vi "I64_Write.vi"(8 "error in (no error)":errorcluster, 9 "Value":i64, 11 "Tag Name":string) -> (0 "error out":errorcluster)   [LabVIEW 2010, in "Current Value Table.lvlib"]
doc: "This VI will write the data associated with a single tag. This VI will always look up the tag index if the name changes, or if index lookup failed previously (resulting in an error). This combines the functionality of the CVT2 VIs for writes and static writes."
uses:
  Current Value Table.lvlib
  FGVs/Tag Memory Methods.ctl
  Type Defs/Memory Commands.ctl
  I64_Type To Enum.vi
  FGVs/CVT Globals.vi
  I64_Memory Block.vi
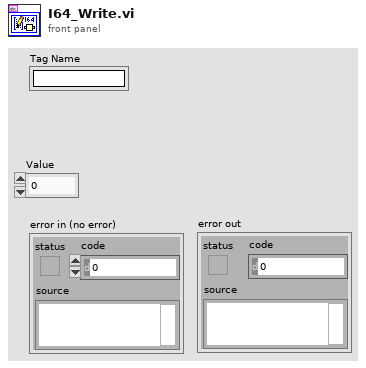
[diagram p1: front panel]
types:
  T1 = typedef "Current Value Table.lvlib/Tag Memory Methods.ctl" = enum16{"Clear", "Read Tag Index", "Read Tag Indices", "Generate Group", "Add Tag", "Overwrite Tag", "Read Description", "Get Stored Tags"}
  T2 = typedef "Current Value Table.lvlib/Data Types.ctl" = enum16{"Double", "Single", "I64", "I32", "I16", "I8", "U64", "U32", "U16", "U8", "String", "Boolean", "Array of U8", "Array of U16", "Array of U32", "Array of U64", "Array of I64", "Array of I32", "Array of I16", "Array of I8", "Array of Double", "Array of Single", "Array of Boolean", "Array of String"}
  T3 = typedef "Current Value Table.lvlib/Memory Commands.ctl" = enum16{"Init", "Add Data", "Read", "Read Group", "Read All", "Write", "Write Group", "Get Size"}
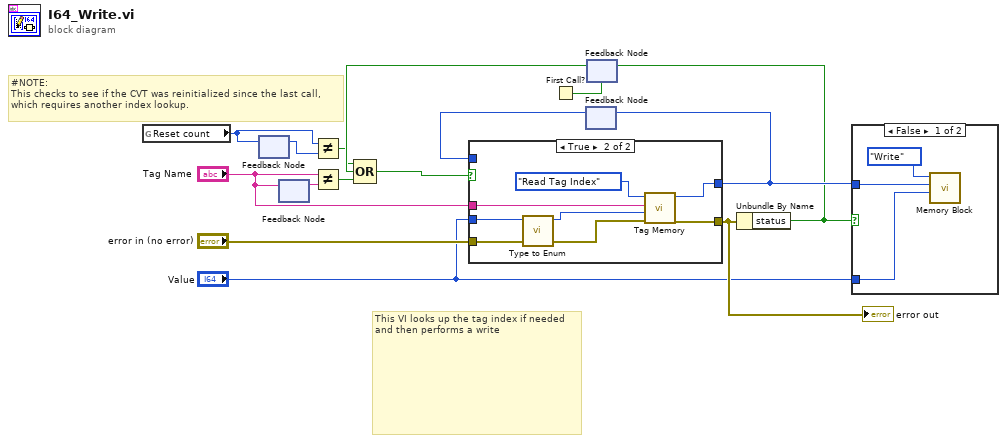
[diagram p0: block diagram]
diagram:
  # "#NOTE:\nThis checks to see if the CVT was reinitialized since the last call,\nwhich requires another index lookup."
  # "This VI looks up the tag index if needed and then performs a write"
  n1 = global read "CVT Globals.vi" "Reset count"() -> (w2:u32)
  n2 = feedback #1() -> (w3:u32)  [unwired: 1 in]
  n3 = feedback-in #1(w2) -> ()
  n4 = feedback #2() -> (w13:string)  [unwired: 1 in]
  n5 = feedback-in #2("Tag Name") -> ()
  n6 = Not Equal?(x=w2, y=w3) -> (x != y?=w1:bool)
  n7 = Not Equal?(x="Tag Name", y=w13) -> (x != y?=w6:bool)
  n8 = First Call?() -> (First Call?: T/F=w5:bool)
  n9 = feedback #3() -> (w12:i32)  [unwired: 1 in]
  n10 = feedback #4(w5) -> (w8:bool)
  n11 = Compound Arithmetic op=OR(w1, w8, w6) -> (w7:bool)
  n12 = case shown="True" w7 {
    tunnel: [w17 w22] -> w9
    tunnel: "error in (no error)" -> [w17 w18]
    tunnel: [w16 w21] -> w15
    tunnel: w12 -> [w16 _]
    tunnel: "Tag Name" -> [_ w20]
    tunnel: "Value" -> [_ w24]
    frame False {
    }
    frame True {
      n13 = call-poly "Type to Enum.vi"("Default"=w24) -> ("Data Type Enum"=w19:T2)  [unwired: 10 in]
      n14 = call "Tag Memory.vi"("error in (no error)"=w18, "Expected Type"=w19, "Tag"=w20, "Method"=Tag_Memory_Methods."Read Tag Index") -> ("error out"=w22:errorcluster, "Index Out"=w21:i32)  [unwired: 2 in, 4 out]
    }
  }
  "error out" <- w9
  n15 = feedback-in #3(w15) -> ()
  n16 = Unbundle By Name(w9) -> ("status"=w10:bool)
  n17 = feedback-in #4(w10) -> ()
  n18 = case shown="False" w10 {
    tunnel: w15 -> [w26 _]
    tunnel: "Value" -> [w25 _]
    frame False {
      n19 = call-poly "Memory Block.vi"("Value"=w25, "Index"=w26, "Method"=Memory_Commands."Write") -> ()  [unwired: 6 in, 3 out]
    }
    frame True {
    }
  }
